vi "innovation covariance.vi"(10 "R":T1=[[0.1]], 11 "Pk|k-1":T1) -> (2 "S_k array":dbl[][](array[numeric]), 3 "S_k":T1)   [LabVIEW 2017]
uses:
  <vilib>/Analysis/Matrix/Datatypes/RealMatrix.ctl
  <vilib>/Analysis/Matrix/NI_Matrix.lvlib
  <vilib>/Analysis/Matrix/Numeric/Multiply/Multiply - RM,RM.vi
  <vilib>/Analysis/Matrix/Numeric/Add/Add - RM,RM.vi
  <vilib>/Analysis/Matrix/Numeric/Conversions/Matrix To Array - RM.vi
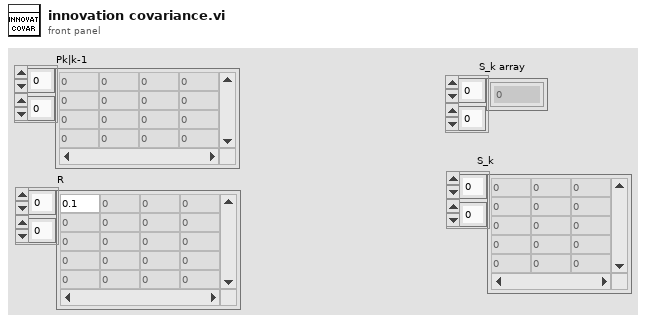
[diagram p1: front panel]
types:
  T1 = typedef "NI_Matrix.lvlib/RealMatrix.ctl" = dbl[][]
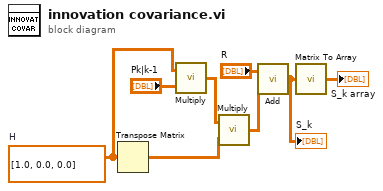
[diagram p0: block diagram]
diagram:
  w1 = T1 [[1.0, 0.0, 0.0]]  # H
  n1 = Transpose Matrix(1:w1) -> (0:w2:T1)
  n2 = call-poly <vilib>:"Multiply.vi"("Real Matrix B"="Pk|k-1", "Real Matrix A"=w1) -> ("A * B"=w8:T1)
  n3 = call-poly <vilib>:"Multiply.vi"("Real Matrix B"=w2, "Real Matrix A"=w8) -> ("A * B"=w7:T1)
  n4 = call-poly <vilib>:"Add.vi"("Real Matrix B"=w7, "Real Matrix A"="R") -> ("A + B"=w5:T1)
  "S_k" <- w5
  n5 = call-poly <vilib>:"Matrix To Array.vi"("Real Matrix"=w5) -> ("Real 2D Array"=→"S_k array":dbl[][])
